vi "Process.vi"(8 "error in":errorcluster, 11 "Example Instrument UI":refnum<class "Instrument.PPMS2 UI.lvclass">) -> (0 "error out":errorcluster, 3 "Example Instrument UI out":refnum<class "Instrument.PPMS2 UI.lvclass">)   [LabVIEW 2016, in "Instrument.PPMS2 UI.lvclass"]
doc: "---------------------------------------------------------------\nJKI State Machine Objects™\nhttp://jki.net/state-machine-objects/\nCopyright (C) 2005-2015, JKI <info@jki.net>\nALL RIGHTS RESERVEDJKI State Machine Objects (SMO) 1.0.0.5\nJKI - JKI\nCopyright (c) 2016, JKI"
uses:
  Instrument.PPMS2 UI.lvclass
  C:/Program Files (x86)/National Instruments/LabVIEW 2016/vi.lib/JKI/JKI SMO/SMO/SMO.lvclass
  C:/Program Files (x86)/National Instruments/LabVIEW 2016/vi.lib/JKI/JKI SMO/SMO.UI/SMO.UI.lvclass
  instrument.PPMS2/Typedefs/Magnet Status--PPMS2--ring.ctl
  instrument.PPMS2/Typedefs/Temperature Status--PPMS2--ring.ctl
  <vilib>/JKI/JKI SMO/SMO/Typedefs/Parent Call--Enum.ctl
  instrument.PPMS2/instrument.PPMS2.lvclass
  C:/Program Files (x86)/National Instruments/LabVIEW 2016/user.lib/LevyLab/Levylab Instruments/SMOs/Instrument/Instrument.lvclass
  Instrument.PPMS2 UI.lvclass/Instrument.PPMS2 UI.ctl
  instrument.PPMS2/Typedefs/getAll--PPMS2--cluster.ctl
  <vilib>/JKI/JKI SMO/SMO.UI/SMO.UI.lvclass
  <vilib>/JKI/JKI SMO/SMO/SMO.lvclass
  <userlib>/LevyLab/Levylab Instruments/SMOs/Instrument/Instrument.lvclass
panel:
  in  "Angle":bool
  in  "Field":bool
  in  "Temperature":bool
  in  "Target Angle (°)":dbl=-0.00643419474363327 format="%_3g"
  in  "Target Field (Oe)":dbl=-0.00643419474363327 format="%_3g"
  in  "Target Temperature (K)":dbl=305.0156 format="%#_5g"
  out "PPMS 2 Temperature Status":T1 items=["TemperatureUnknown"=0, "Stable"=1, "Tracking"=2, "Near"=5, "Chasing"=6, "Filling"=7, "Standby"=10, "Disabled"=13, "ImpedanceNotFunction"=14, "TempFailure"=15]
  out "PPMS 2 Magnet Status":T2=1 items=["MagnetUnknown"=0, "StablePersistent"=1, "WarmingSwitch"=2, "CoolingSwitch"=3, "StableDriven"=4, "Iterating"=5, "Charging"=6, "Discharging"=7, "CurrentError"=8, "MagnetFailure"=15]
  out "Helium Level (%)":dbl=86.7
  out "Position (°)":dbl=90.002
  out "Field (Oe)":dbl=-0.00643419474363327 format="%_3g"
  out "Temperature(K)":dbl=305.0156 format="%#_5g"
  in  "update time (ms)":u32=200
  in  "STOP":bool
  # "PPMS 2 Monitor"
  # "SMO UI Template"
  # "For instructions on how to use the JKI State Machine Objects, examples and video tutorials, visit:\nhttp://jki.net/state-machine-objects/\n\nJKI State Machine Objects™\nhttp://jki.net/state-machine-objects/\nCopyright (C) 2005-2015, JKI <info@jki.net>\nALL RIGHTS RESERVED"
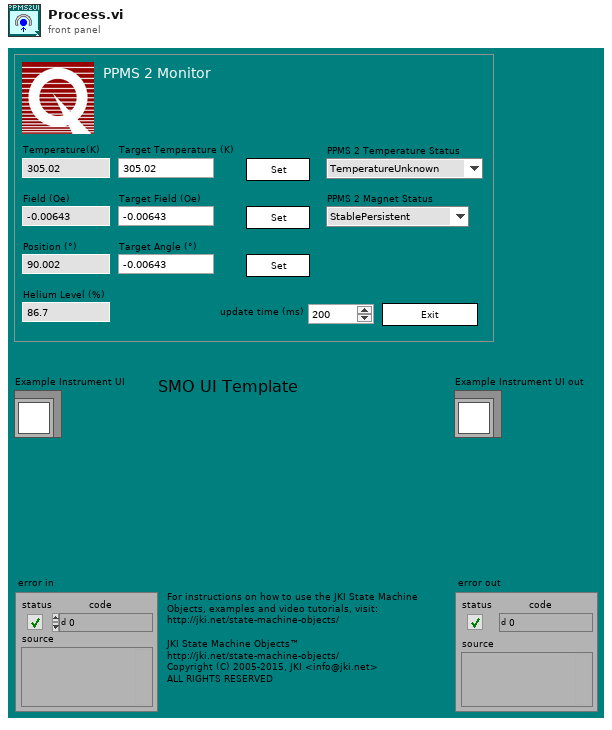
[diagram p1: front panel]
types:
  T1 = typedef "instrument.PPMS2.lvclass/Temperature Status--PPMS2--ring.ctl" = i32
  T2 = typedef "instrument.PPMS2.lvclass/Magnet Status--PPMS2--ring.ctl" = i32
  T3 = typedef "SMO.lvclass/Parent Call--Enum.ctl" = enum16{"Allows parent to run", "Does not request parent to run"}
  T4 = enum32{"invalid app kind", "Development System", "Run Time System", "Student Edition", "Embedded LabVIEW", "Evaluation", "Custom"}
  T5 = enum32{"Invalid", "Standard", "Closed", "Hidden", "Minimized", "Maximized"}
  T6 = typedef "instrument.PPMS2.lvclass/getAll--PPMS2--cluster.ctl" = cluster{"PPMS 2 Helium Level":dbl, "PPMS 2 Temperature":dbl, "PPMS 2 Temperature Status":T1, "PPMS 2 Magnetic Field":dbl, "PPMS 2 Magnet Status":T2, "PPMS 2 Position":dbl}
  T7 = cluster{"Core":cluster{"Current VI Reference":refnum<vi>, "Close Panel on Exit?":bool, "error":errorcluster}, "Self Reference":refnum<class "Instrument.PPMS2 UI.lvclass">, "instrument.PPMS2":refnum<class "instrument.PPMS2.lvclass">, "Data Send":variant, "Data Receive":variant}
  T8 = cluster{"Current VI Reference":refnum<vi>, "Close Panel on Exit?":bool, "error":errorcluster}
  T9 = typedef "SMO.lvclass/Protected Events.ctl" = cluster{"StopProcesses":refnum<user-event>, "AbortProcesses":refnum<user-event>, "Config Changed":refnum<user-event>, "Dependency":refnum<user-event>}
  T10 = typedef "Instrument.lvclass/PublicEvents--Cluster.ctl" = cluster{"MessageFromProcess":refnum<user-event>}
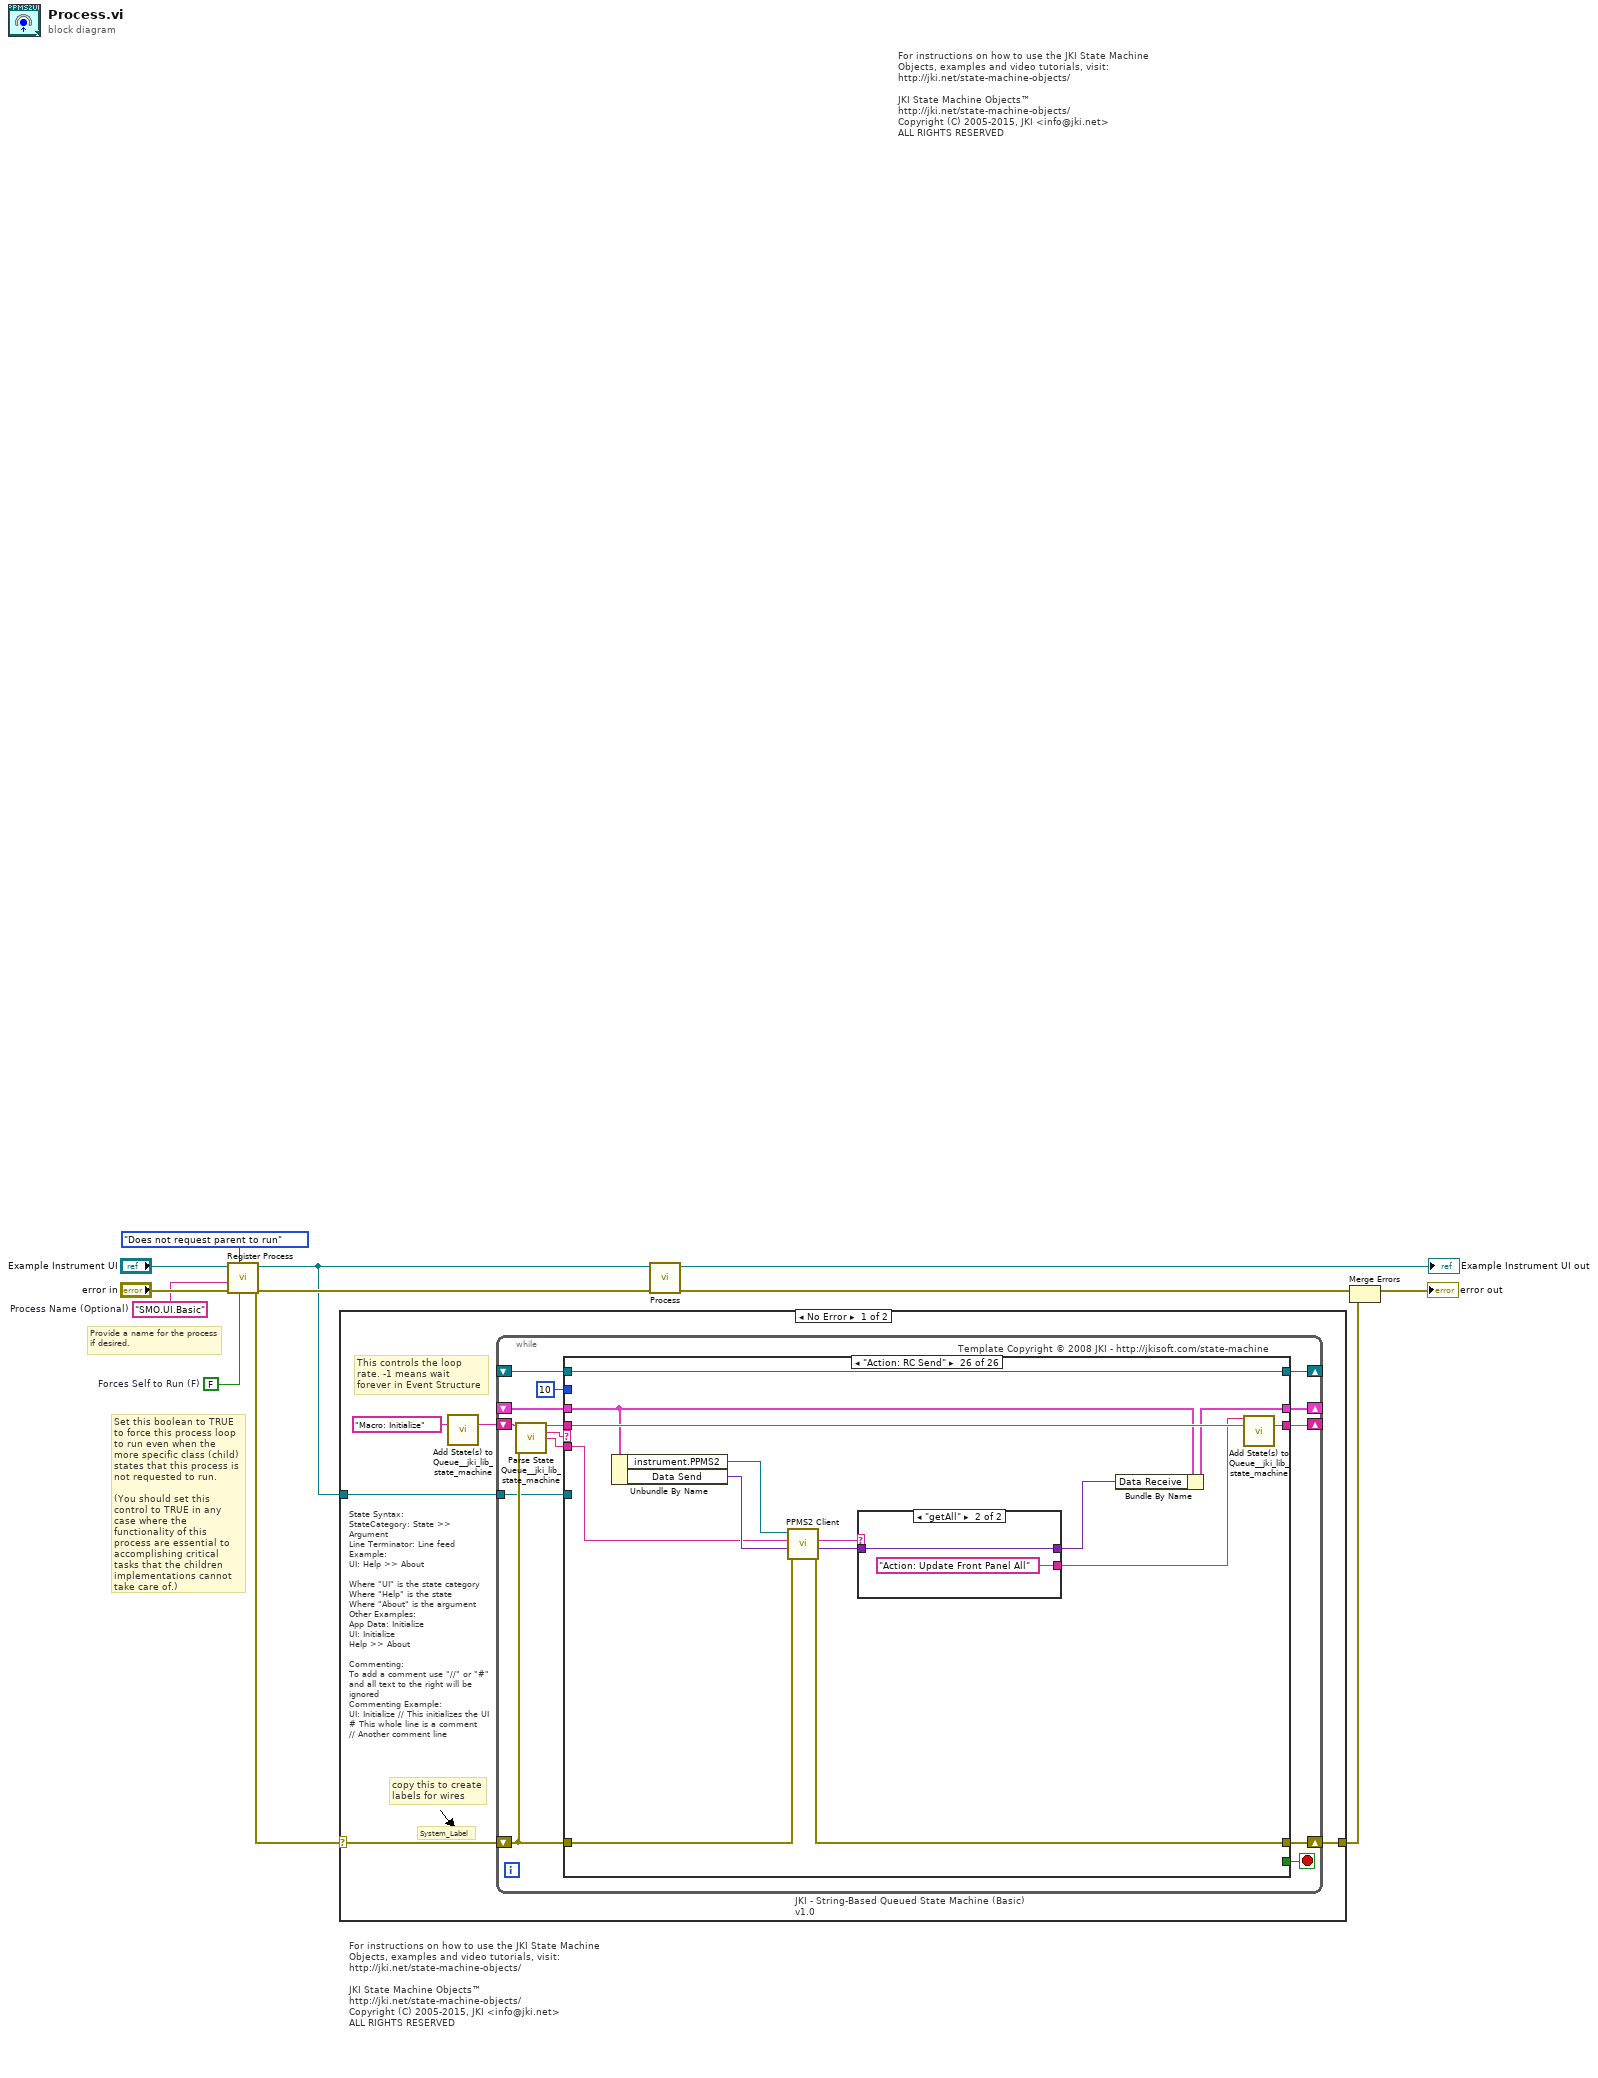
[diagram p0: block diagram]
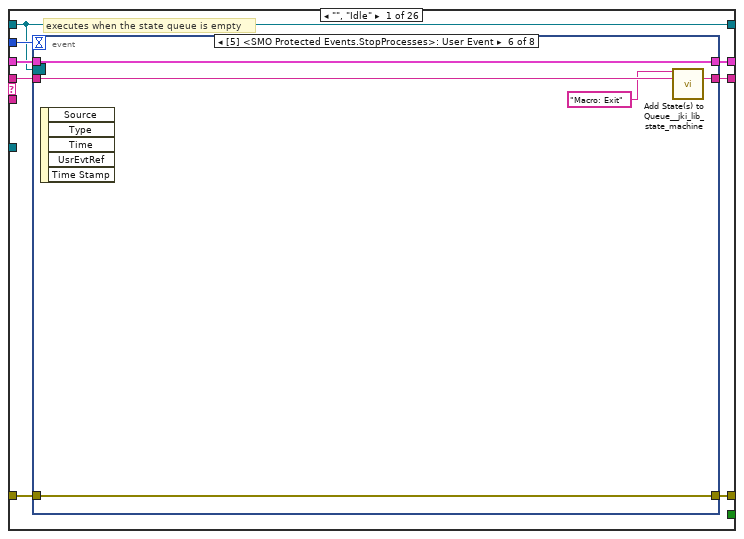
[diagram p2: hidden frame]
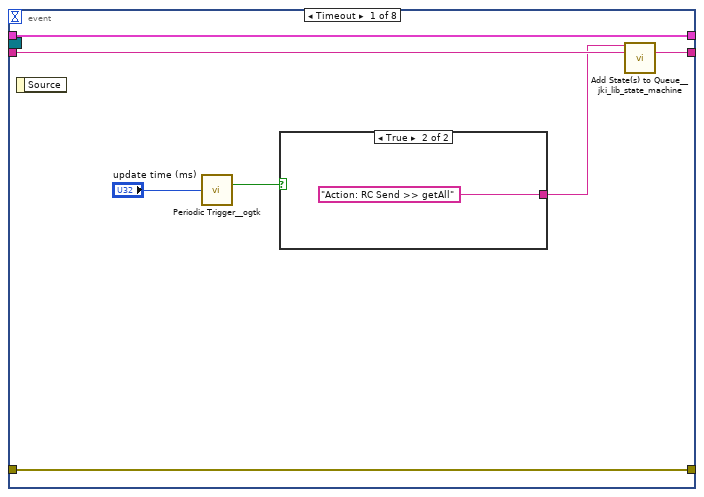
[diagram p3: hidden frame]
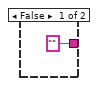
[diagram p4: hidden frame]
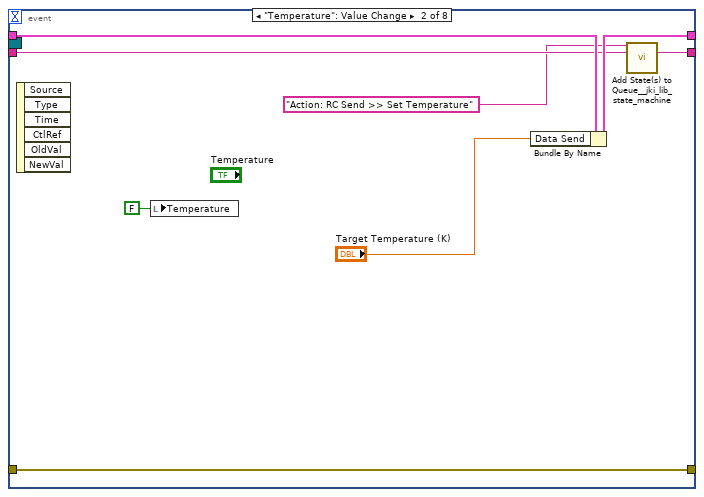
[diagram p5: hidden frame]
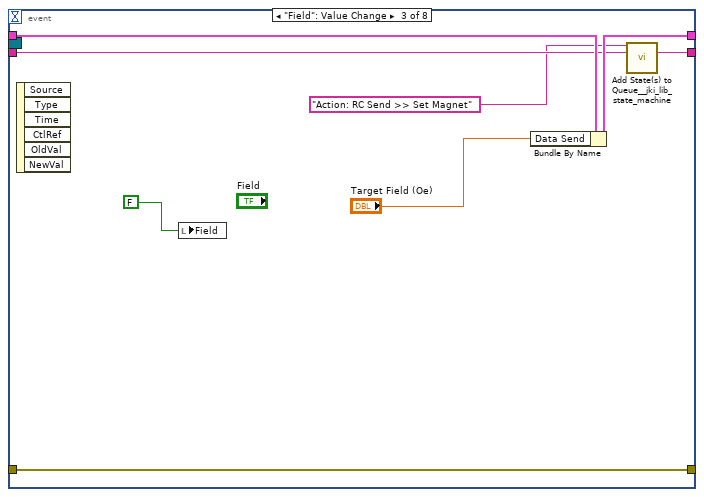
[diagram p6: hidden frame]
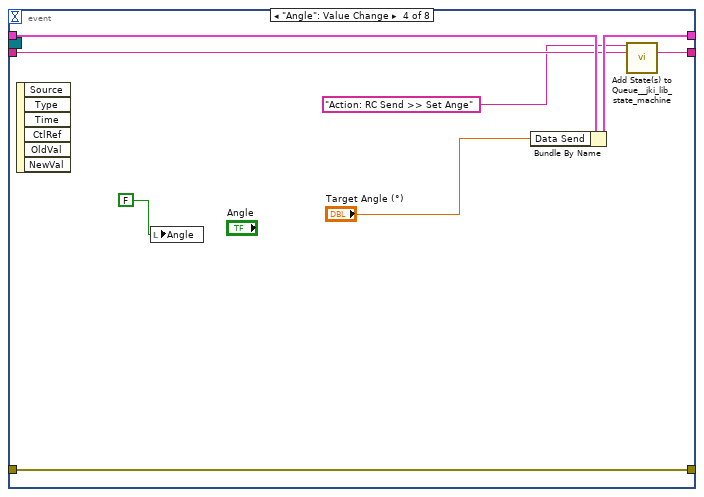
[diagram p7: hidden frame]
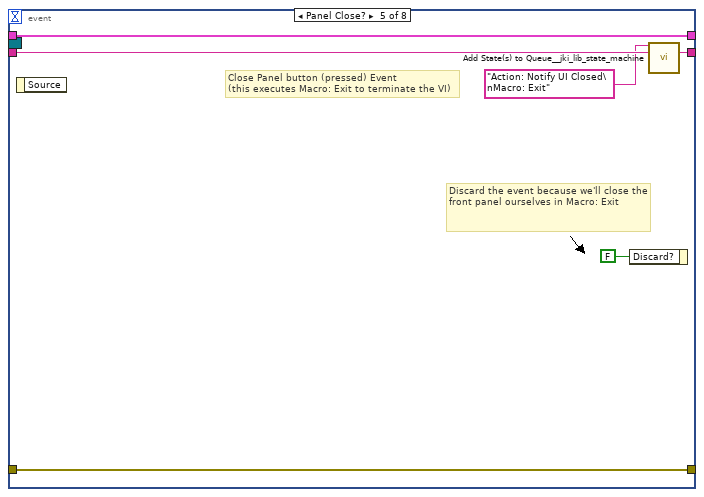
[diagram p8: hidden frame]
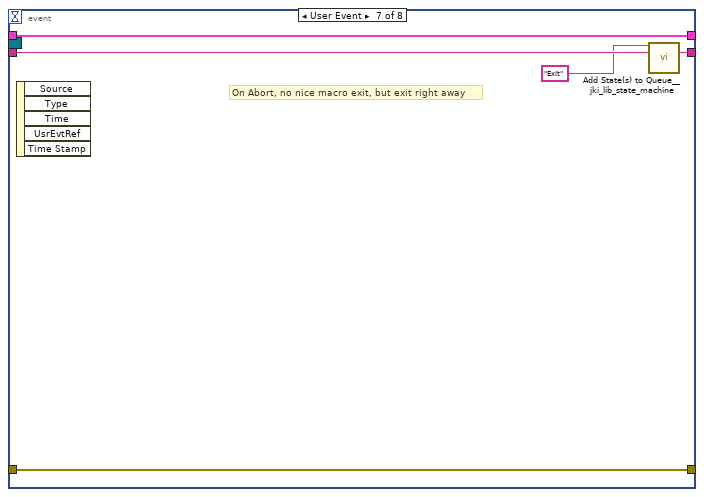
[diagram p9: hidden frame]
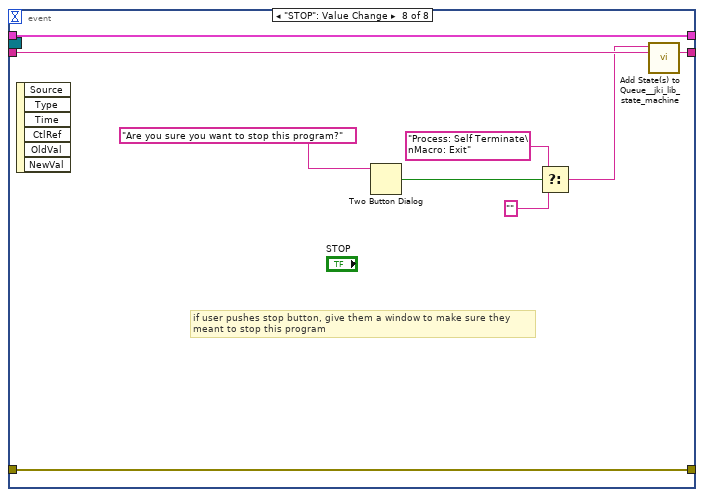
[diagram p10: hidden frame]
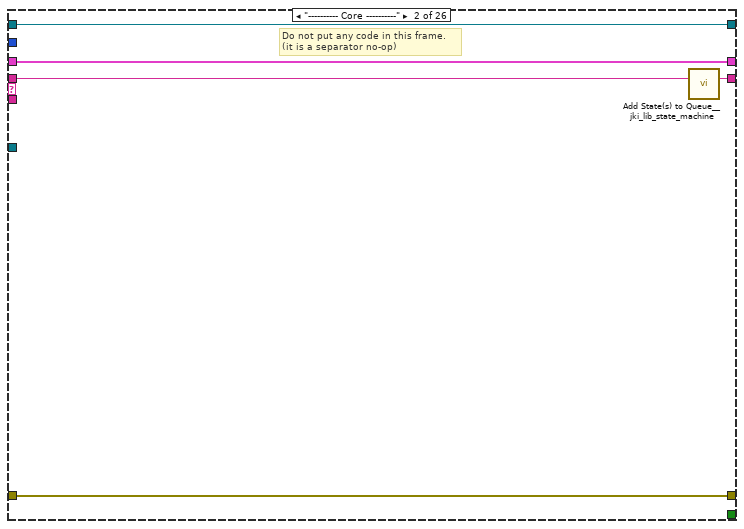
[diagram p11: hidden frame]
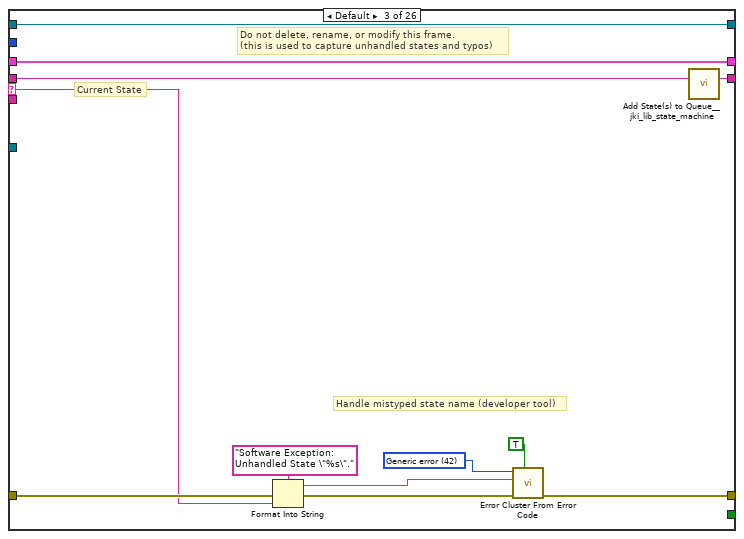
[diagram p12: hidden frame]
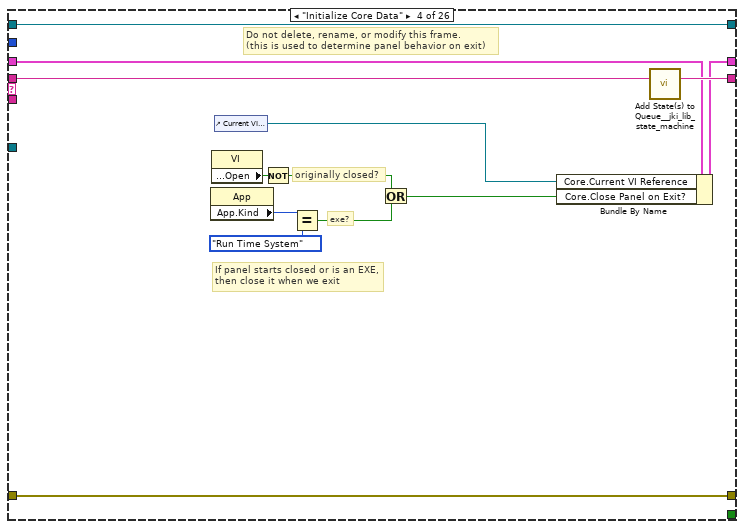
[diagram p13: hidden frame]
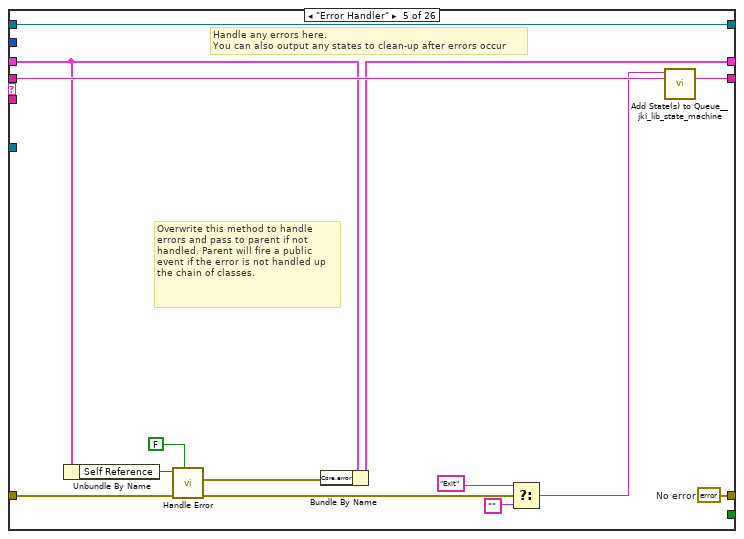
[diagram p14: hidden frame]
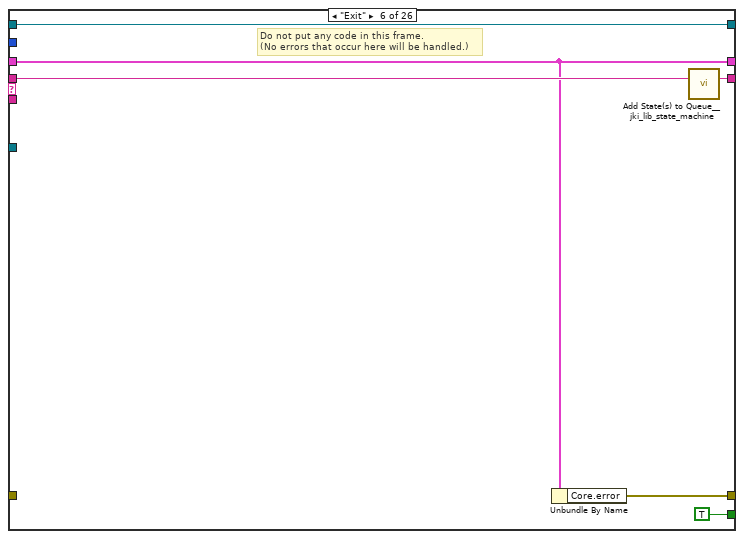
[diagram p15: hidden frame]
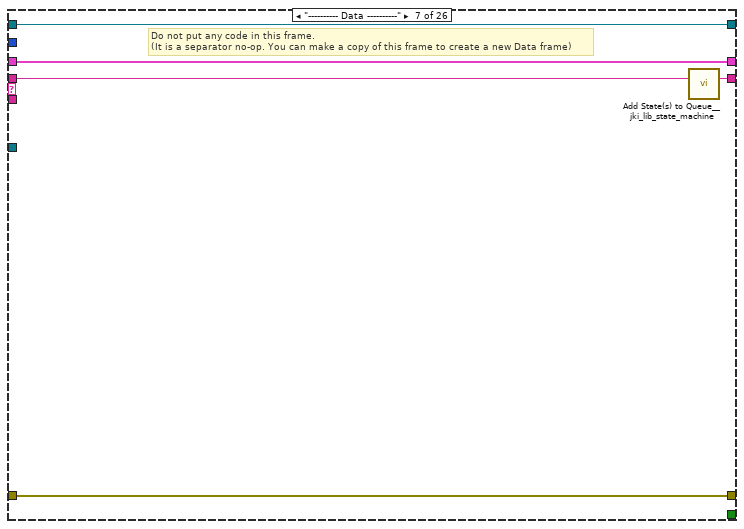
[diagram p16: hidden frame]
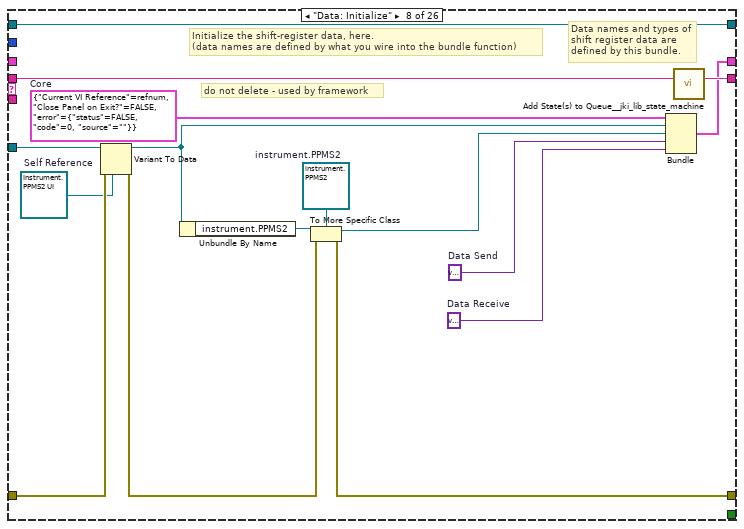
[diagram p17: hidden frame]
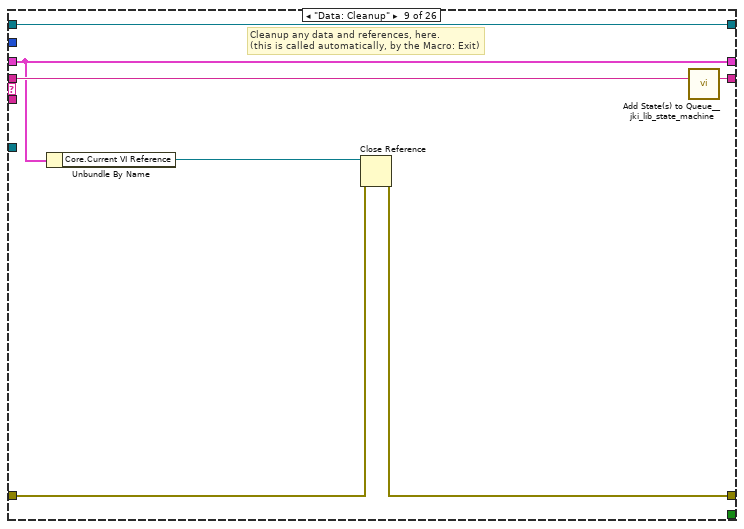
[diagram p18: hidden frame]
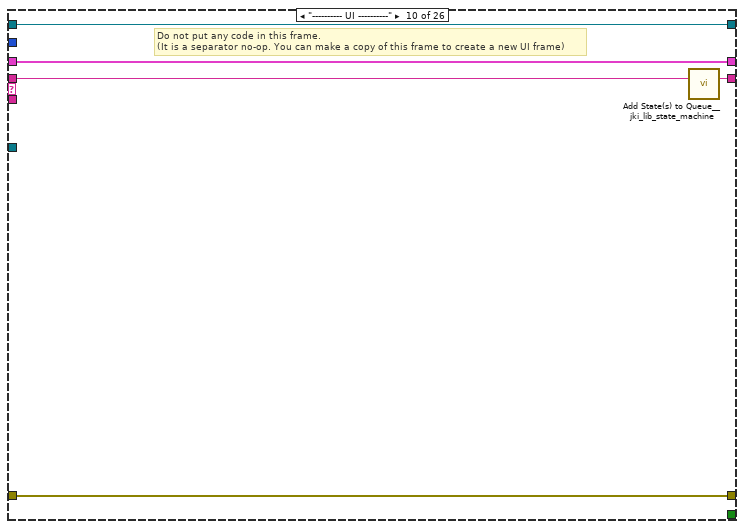
[diagram p19: hidden frame]
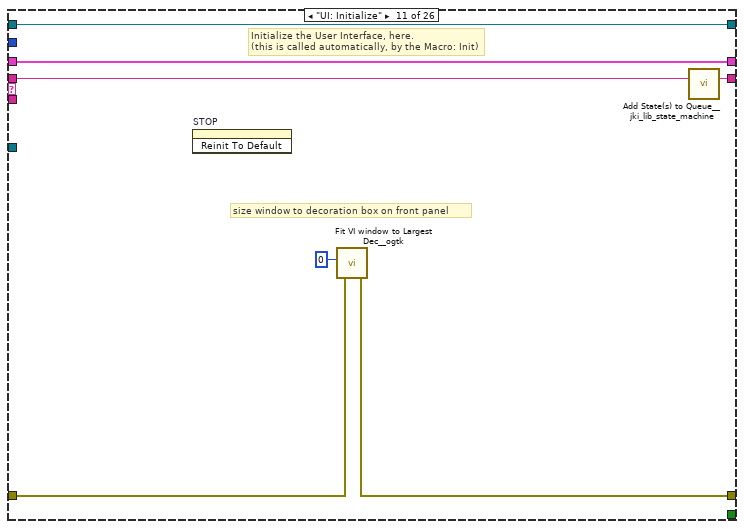
[diagram p20: hidden frame]
diagram:
  w2 = FALSE  # Forces Self to Run (F)
  w1 = "SMO.UI.Basic"  # Process Name (Optional)
  # "For instructions on how to use the JKI State Machine Objects, examples and video tutorials, visit:\nhttp://jki.net/state-machine-objects/\n\nJKI State Machine Objects™\nhttp://jki.net/state-machine-objects/\nCopyright (C) 2005-2015, JKI <info@jki.net>\nALL RIGHTS RESERVED"
  # "Provide a name for the process\nif desired."
  # "Set this boolean to TRUE to force this process loop to run even when the more specific class (child) states that this process is not requested to run.\n\n(You should set this control to TRUE in any case where the functionality of this process are essential to accomplishing critical tasks that the children implementations cannot take care of.)"
  # "For instructions on how to use the JKI State Machine Objects, examples and video tutorials, visit:\nhttp://jki.net/state-machine-objects/\n\nJKI State Machine Objects™\nhttp://jki.net/state-machine-objects/\nCopyright (C) 2005-2015, JKI <info@jki.net>\nALL RIGHTS RESERVED"
  n1 = call <vilib>:"Register Process.vi"("Forces Self to Run (F)"=w2, "Parent Call"=Parent_Call--Enum."Does not request parent to run", "error in (no error)"="error in", "Process Name (optional)"=w1, "SMO"="Example Instrument UI") -> ("error out"=w8:errorcluster, "SMO out"=w7:refnum<class "Instrument.PPMS2 UI.lvclass">)  [unwired: 5 in]
  n2 = case shown="No Error" w8 {
    selector: w8 -> [w13 w359]
    tunnel: w7 -> [w14 _]
    tunnel: [w12 w359] -> w4
    frame No Error {
      # "State Syntax:\nStateCategory: State >> Argument\nLine Terminator: Line feed\nExample:\nUI: Help >> About\n\nWhere \"UI\" is the state category\nWhere \"Help\" is the state\nWhere \"About\" is the argument\nOther Examples:\nApp Data: Initialize\nUI: Initialize\nHelp >> About\n\nCommenting:\nTo add a comment use \"//\" or \"#\" and all text to the right will be ignored\nCommenting Example:\nUI: Initialize // This initializes the UI\n# This whole line is a comment\n// Another comment line"
      # "copy this to create labels for wires"
      # "This controls the loop rate. -1 means wait forever in Event Structure"
      # "System_Label"
      n3 = call <vilib>:"Add State(s) to Queue__jki_lib_state_machine.vi"("State(s) in (\"\")"="Macro: Initialize") -> ("States Out"=w16:string)  [unwired: 14 in]
      n4 = while "JKI - String-Based Queued State Machine (Basic) v1.0" {
        shift-right: [w23] -> _
        shift-left: _ -> [w22]
        shift-right: [w26] -> w12
        shift-left: w13 -> [w20]
        shift-right: [w25] -> _
        shift-left: w16 -> [w27]
        tunnel: w14 -> [w19]
        shift-right: [w18] -> _
        shift-left: _ -> [w17]
        stop <- w24 stop-if-true
        # "Template Copyright © 2008 JKI - http://jkisoft.com/state-machine"
        n5 = call <vilib>:"Parse State Queue__jki_lib_state_machine.vi"("State Queue"=w27, "Error In (no error)"=w20) -> ("Remaining States"=w29:string, "Current State"=w30:string, "Arguments"=w28:string)  [unwired: 11 in]
        n6 = case shown="\"Action: RC Send\"" w30 {
          selector: w30 -> [_ _ w103 _ _ _ _ _ _ _ _ _ _ _ _ _ _ _ _ _ _ _ _ _ _ _]
          tunnel: w29 -> [w38 w101 w107 w126 w140 w146 w151 w167 w174 w179 w186 w193 w209 w241 w250 w264 w269 w280 w287 w292 w305 w311 w318 w325 w340 w354]
          tunnel: w28 -> [_ _ _ _ _ _ _ _ _ _ _ w187 w203 _ _ _ _ _ _ _ _ _ _ _ _ w346]
          tunnel: w22 -> [w36 w98 w105 w117 w128 w142 w148 _ w170 w176 w184 w191 w205 w238 w246 w255 w266 w277 w282 w289 w303 w309 w314 w321 w337 w351]
          tunnel: [w35 w99 w109 w123 w133 w141 w149 w153 w171 w177 w181 w188 w206 w239 w248 w262 w267 w271 w283 w290 w298 w306 w315 w319 w335 w344] -> w26
          tunnel: w20 -> [w34 w99 w108 w123 w129 _ w149 w164 w168 w177 w182 w189 w207 w239 w248 w262 w267 w272 w284 w290 w300 w307 w315 w320 w336 w345]
          tunnel: [w37 w100 w106 w125 w139 w145 w150 w166 w173 w178 w185 w192 w208 w240 w249 w263 w268 w279 w286 w291 w304 w310 w317 w324 w339 w353] -> w25
          tunnel: [_ _ _ _ _ TRUE _ _ _ _ _ _ _ _ _ _ _ _ _ _ _ _ _ _ _ _] -> w24
          tunnel: [w33 w98 w105 w124 w131 w142 w148 w165 w170 w176 w184 w191 w205 w238 w246 w255 w266 w277 w282 w289 w303 w309 w313 w321 w337 w350] -> w23
          tunnel: 10 ("Timeout") -> [w32 _ _ _ _ _ _ _ _ _ _ _ _ _ _ _ _ _ _ _ _ _ _ _ _ _]
          tunnel: w19 -> [_ _ _ _ _ _ _ w162 _ _ _ _ _ _ _ _ _ _ _ _ _ _ _ _ _ _]
          tunnel: [w31 w97 w102 w114 w138 w143 w147 w161 w169 w175 w183 w190 w202 w237 w247 w256 w265 w278 w285 w288 w302 w308 w316 w323 w338 w352] -> w18
          tunnel: w17 -> [w31 w97 w102 w114 w138 w143 w147 w161 w169 w175 w183 w190 w202 w237 w247 w256 w265 w278 w285 w288 _ w308 w316 w323 w338 w352]
          frame "", "Idle" {
            # "executes when the state queue is empty"
            n7 = event shown="[5] <SMO Protected Events.StopProcesses>: User Event" {
              selector: w31 -> [_ _ _ _ _ _ _ _]
              dyn-events: _ -> [_ _ _ _ _ _ _ _]
              timeout: w32 -> [_ _ _ _ _ _ _ _]
              tunnel: w38 -> [w45 w51 w59 w67 w77 w82 w87 w96]
              tunnel: [w44 w54 w62 w70 w76 w81 w86 w95] -> w37
              tunnel: w36 -> [w42 w53 w61 w69 w73 w79 w84 w93]
              tunnel: [w43 w55 w63 w71 w72 w80 w85 w94] -> w35
              tunnel: w34 -> [w43 w55 w63 w71 w72 w80 w85 w94]
              tunnel: [w42 w52 w60 w68 w73 w79 w84 w93] -> w33
              event Timeout {
                n8 = event-data() -> ()  [unwired: 1 in, 1 out]
                n9 = call <userlib>:"Periodic Trigger__ogtk.vi"("time (ms)"="update time (ms)") -> ("Triggered"=w41:bool)  [unwired: 12 in, 2 out]
                n10 = case shown="True" w41 {
                  tunnel: ["" "Action: RC Send >> getAll"] -> w39
                  frame False {
                  }
                  frame True {
                  }
                }
                n11 = call <vilib>:"Add State(s) to Queue__jki_lib_state_machine.vi"("State(s) in Front (\"\")"=w39, "State(s) in (\"\")"=w45) -> ("States Out"=w44:string)  [unwired: 13 in]
              }
              event "Temperature": Value Change {
                n12 = event-data() -> ()  [unwired: 1 in, 6 out]
                n13 = local write "Temperature"(FALSE ("Temperature")) -> ()
                n14 = Bundle By Name(cluster=w53, "Data Send"="Target Temperature (K)") -> (w52:T7)
                n15 = call <vilib>:"Add State(s) to Queue__jki_lib_state_machine.vi"("State(s) in Front (\"\")"="Action: RC Send >> Set Temperature" ("State(s) in Front (\"\")"), "State(s) in (\"\")"=w51) -> ("States Out"=w54:string)  [unwired: 13 in]
              }
              event "Field": Value Change {
                n16 = event-data() -> ()  [unwired: 1 in, 6 out]
                n17 = local write "Field"(FALSE ("Field")) -> ()
                n18 = Bundle By Name(cluster=w61, "Data Send"="Target Field (Oe)") -> (w60:T7)
                n19 = call <vilib>:"Add State(s) to Queue__jki_lib_state_machine.vi"("State(s) in Front (\"\")"="Action: RC Send >> Set Magnet" ("State(s) in Front (\"\")"), "State(s) in (\"\")"=w59) -> ("States Out"=w62:string)  [unwired: 13 in]
              }
              event "Angle": Value Change {
                n20 = event-data() -> ()  [unwired: 1 in, 6 out]
                n21 = local write "Angle"(FALSE ("Angle")) -> ()
                n22 = Bundle By Name(cluster=w69, "Data Send"="Target Angle (°)") -> (w68:T7)
                n23 = call <vilib>:"Add State(s) to Queue__jki_lib_state_machine.vi"("State(s) in Front (\"\")"="Action: RC Send >> Set Ange" ("State(s) in Front (\"\")"), "State(s) in (\"\")"=w67) -> ("States Out"=w70:string)  [unwired: 13 in]
              }
              event Panel Close? {
                # "Discard the event because we'll close the front panel ourselves in Macro: Exit"
                # "Close Panel button (pressed) Event\n(this executes Macro: Exit to terminate the VI)"
                n24 = event-data() -> ()  [unwired: 1 in, 1 out]
                n25 = event-data("Discard?"=FALSE) -> ()  [unwired: 1 in, 1 out]
                n26 = call <vilib>:"Add State(s) to Queue__jki_lib_state_machine.vi"("State(s) in Front (\"\")"="Action: Notify UI Closed\nMacro: Exit", "State(s) in (\"\")"=w77) -> ("States Out"=w76:string)  [unwired: 13 in]
              }
              event User Event {
                n27 = event-data() -> ()  [unwired: 1 in, 5 out]
                n28 = call <vilib>:"Add State(s) to Queue__jki_lib_state_machine.vi"("State(s) in Front (\"\")"="Macro: Exit", "State(s) in (\"\")"=w82) -> ("States Out"=w81:string)  [unwired: 13 in]
              }
              event User Event {
                # "On Abort, no nice macro exit, but exit right away"
                n29 = event-data() -> ()  [unwired: 1 in, 5 out]
                n30 = call <vilib>:"Add State(s) to Queue__jki_lib_state_machine.vi"("State(s) in Front (\"\")"="Exit", "State(s) in (\"\")"=w87) -> ("States Out"=w86:string)  [unwired: 13 in]
              }
              event "STOP": Value Change {
                # "if user pushes stop button, give them a window to make sure they\nmeant to stop this program"
                n31 = event-data() -> ()  [unwired: 1 in, 6 out]
                n32 = Two Button Dialog(message="Are you sure you want to stop this program?") -> (T button?=w92:bool)  [unwired: 2 in]
                n33 = Select(t="Process: Self Terminate\nMacro: Exit", s=w92, f="") -> (s? t:f=w88:string)
                n34 = call <vilib>:"Add State(s) to Queue__jki_lib_state_machine.vi"("State(s) in Front (\"\")"=w88, "State(s) in (\"\")"=w96) -> ("States Out"=w95:string)  [unwired: 13 in]
              }
            }
          }
          frame "---------- Core ----------" {
            # "Do not put any code in this frame.\n(it is a separator no-op)"
            n35 = call <vilib>:"Add State(s) to Queue__jki_lib_state_machine.vi"("State(s) in (\"\")"=w101) -> ("States Out"=w100:string)  [unwired: 14 in]
          }
          frame Default {
            w112 = 42 items=["No error", "Argument error", "Memory is full", "Out of zone", "End of file", "File already open", "Generic file I/O error", "File not found", "File permission error", "Disk is full", "Duplicate path", "Too many files open", "System feature not enabled", "Resource file not found", "Cannot add resource", "Resource not found", "Image not found", "Image memory error", "Pen does not exist", "Config type invalid", "Config token not found", "Config parse error", "Config memory error", "Bad external code format", "Bad external code offset", "External code not present", "Null window", "Destroy window error", "Null menu", "Print aborted", "Bad print record", "Print driver error", "Windows error during printing", "Memory error during printing", "Print dialog error", "Generic print error", "Invalid device refnum", "Device not found", "Device parameter error", "Device unit error", "Cannot open device", "Device call aborted", "Generic error", "Cancelled by user", "Object ID too low", "Object ID too high", "Object not in heap", "Unknown heap", "Unknown object (invalid DefProc)", "Unknown object (DefProc not in table)", "Message out of range", "Invalid (null) method", "Unknown message", "Manager call not supported", "Bad address", "Network operation in progress", "Network operation timed out", "Connection is busy", "Network attribute not supported", "Network error", "Address in use", "System out of memory", "Connection aborted", "Connection refused", "Not connected", "Already connected", "Connection closed", "Initialization error (interapplication manager)", "Bad occurrence", "Wait on unbound occurrence handler", "Occurrence queue overflow", "Datalog type conflict", "Unused", "Unrecognized type (interapplication manager)", "Memory corrupt", "Failed to make temporary DLL", "Old CIN version", "Drag socket not found", "Failed to load drop-object", "Failed to register OLE object", "Failed to release OLE object", "Format specifier type mismatch", "Unknown format specifier", "Too few format specifiers", "Too many format specifiers", "Scan failed", "Newer CIN version", "Error converting to variant", "Runtime menu error", "Password tampered", "Variant attribute not found", "Incompatible variant data type", "Event data is not available", "Event Store is not present", "Occurrence is not found", "Event Queue is not created", "Event info is not available", "Refnum passed is NULL", "Error retrieving Class GUID", "Error retrieving CoClass GUID", "Error retrieving TypeLib GUID.", "Bad built application magic bytes.", "Specific driver is different from the specific driver associated with the Logical Name.", "There is no session opened to the class driver.", "Max Error", "MAX - Error with config objects", "MAX - Error loading configuration", "MAX - Group not supported"]
            # "Current State"
            # "Do not delete, rename, or modify this frame.\n(this is used to capture unhandled states and typos)"
            # "Handle mistyped state name (developer tool)"
            n36 = Format Into String(format string="Software Exception: Unhandled State \"%s\"." ("message"), error in=w108, w103) -> (resulting string=w111:string, error out=w110:errorcluster)  [unwired: 1 in]
            n37 = call <vilib>:"Error Cluster From Error Code.vi"("show call chain? (False)"=TRUE, "error in (no error)"=w110, "error message (\"\")"=w111, "error code (0)"=w112) -> ("error out"=w109:errorcluster)  [unwired: 5 in]
            n38 = call <vilib>:"Add State(s) to Queue__jki_lib_state_machine.vi"("State(s) in (\"\")"=w107) -> ("States Out"=w106:string)  [unwired: 14 in]
          }
          frame "Initialize Core Data" {
            # "Do not delete, rename, or modify this frame.\n(this is used to determine panel behavior on exit)"
            # "originally closed?"
            # "exe?"
            # "If panel starts closed or is an EXE, then close it when we exit"
            n39 = property class="App"() -> ("App.Kind"=w121:T4)  [unwired: 2 in, 2 out]
            n40 = property class="VI"() -> ("Front Panel.Open"=w122:bool)  [unwired: 2 in, 2 out]
            n41 = control-ref of="Current VI Reference"() -> (w115:refnum<vi>)
            n42 = Not(x=w122) -> (.not. x?=w119:bool)
            n43 = Equal?(x=w121, y=T4."Run Time System" ("Application:Kind")) -> (x = y?=w118:bool)
            n44 = Or(x=w119, y=w118) -> (x .or. y?=w116:bool)
            n45 = Bundle By Name(cluster=w117, "Core.Current VI Reference"=w115, "Core.Close Panel on Exit?"=w116) -> (w124:T7)
            n46 = call <vilib>:"Add State(s) to Queue__jki_lib_state_machine.vi"("State(s) in (\"\")"=w126) -> ("States Out"=w125:string)  [unwired: 14 in]
          }
          frame "Error Handler" {
            w133 = errorcluster {"status"=FALSE, "code"=0, "source"=""}  # No error
            # "Overwrite this method to handle errors and pass to parent if not handled. Parent will fire a public event if the error is not handled up the chain of classes."
            # "Handle any errors here.\nYou can also output any states to clean-up after errors occur"
            n47 = Unbundle By Name(w128) -> ("Self Reference"=w137:refnum<class "Instrument.PPMS2 UI.lvclass">)
            n48 = call-dynamic "Handle Error.vi"("Stop on Unhandled Error (T)"=FALSE, "error in"=w129, "SMO"=w137) -> ("handling error"=w127:errorcluster, "Unhandled error"=w132:errorcluster)  [unwired: 6 in, 1 out]
            n49 = Bundle By Name(cluster=w128, "Core.error"=w132) -> (w131:T7)
            n50 = Select(t="Exit", s=w127, f="") -> (s? t:f=w134:string)
            n51 = call <vilib>:"Add State(s) to Queue__jki_lib_state_machine.vi"("State(s) in Front (\"\")"=w134, "State(s) in (\"\")"=w140) -> ("States Out"=w139:string)  [unwired: 13 in]
          }
          frame "Exit" {
            # "Do not put any code in this frame.\n(No errors that occur here will be handled.)"
            n52 = Unbundle By Name(w142) -> ("Core.error"=w141:errorcluster)
            n53 = call <vilib>:"Add State(s) to Queue__jki_lib_state_machine.vi"("State(s) in (\"\")"=w146) -> ("States Out"=w145:string)  [unwired: 14 in]
          }
          frame "---------- Data ----------" {
            # "Do not put any code in this frame.\n(It is a separator no-op. You can make a copy of this frame to create a new Data frame)"
            n54 = call <vilib>:"Add State(s) to Queue__jki_lib_state_machine.vi"("State(s) in (\"\")"=w151) -> ("States Out"=w150:string)  [unwired: 14 in]
          }
          frame "Data: Initialize" {
            w152 = variant  # Data Receive
            w157 = refnum<class "instrument.PPMS2.lvclass"> refnum  # instrument.PPMS2
            w158 = variant  # Data Send
            w160 = T8 {"Current VI Reference"=refnum, "Close Panel on Exit?"=FALSE, "error"={"status"=FALSE, "code"=0, "source"=""}}  # Core
            w163 = refnum<class "Instrument.PPMS2 UI.lvclass"> refnum  # Self Reference
            # "do not delete - used by framework"
            # "Data names and types of shift register data are defined by this bundle."
            # "Initialize the shift-register data, here.\n(data names are defined by what you wire into the bundle function)"
            n55 = Variant To Data(error in=w164, type=w163, Variant=w162) -> (data=w159:refnum<class "Instrument.PPMS2 UI.lvclass">, error out=w154:errorcluster)
            n56 = Unbundle By Name(w159) -> ("instrument.PPMS2"=w156:refnum<class "instrument.PPMS2.lvclass">)
            n57 = To More Specific Class(target class=w157, reference=w156, error in=w154) -> (specific class reference=w155:refnum<class "instrument.PPMS2.lvclass">, error out=w153:errorcluster)
            n58 = Bundle("Core"=w160, "Self Reference"=w159, "instrument.PPMS2"=w155, "Data Send"=w158, "Data Receive"=w152) -> (w165:T7)  [unwired: 1 in]
            n59 = call <vilib>:"Add State(s) to Queue__jki_lib_state_machine.vi"("State(s) in (\"\")"=w167) -> ("States Out"=w166:string)  [unwired: 14 in]
          }
          frame "Data: Cleanup" {
            # "Cleanup any data and references, here.\n(this is called automatically, by the Macro: Exit)"
            n60 = Unbundle By Name(w170) -> ("Core.Current VI Reference"=w172:refnum<vi>)
            n61 = Close Reference(reference=w172, error in (no error)=w168) -> (error out=w171:errorcluster)
            n62 = call <vilib>:"Add State(s) to Queue__jki_lib_state_machine.vi"("State(s) in (\"\")"=w174) -> ("States Out"=w173:string)  [unwired: 14 in]
          }
          frame "---------- UI ----------" {
            # "Do not put any code in this frame.\n(It is a separator no-op. You can make a copy of this frame to create a new UI frame)"
            n63 = call <vilib>:"Add State(s) to Queue__jki_lib_state_machine.vi"("State(s) in (\"\")"=w179) -> ("States Out"=w178:string)  [unwired: 14 in]
          }
          frame "UI: Initialize" {
            # "size window to decoration box on front panel"
            # "Initialize the User Interface, here.\n(this is called automatically, by the Macro: Init)"
            n64 = invoke on="STOP" class="Bool (strict)" method="Reinit To Default"() -> ()  [unwired: 3 in, 3 out]
            n65 = call <userlib>:"Fit VI window to Largest Dec__ogtk.vi"("error in (no error)"=w182, "border spacing (2 px)"=0) -> ("error out"=w181:errorcluster)  [unwired: 4 in, 1 out]
            n66 = call <vilib>:"Add State(s) to Queue__jki_lib_state_machine.vi"("State(s) in (\"\")"=w186) -> ("States Out"=w185:string)  [unwired: 14 in]
          }
          frame "UI: Cursor Set" {
            # "Argument"
            # "Initialize the User Interface, here.\n(this is called automatically, by the Macro: Init)"
            n67 = disable-structure shown="Default" {
              disable-tunnel: w189 -> [w194 w197]
              disable-tunnel: [w194 w196] -> w188
              disable-tunnel: w187 -> [_ w195]
              frame condition #0 {
              }
              frame condition #1 (active) {
                n68 = case shown="\"Busy\"" w195 {
                  tunnel: w197 -> [w199 w201]
                  tunnel: [w198 w200] -> w196
                  frame "Idle", Default {
                    n69 = call <vilib>:"Unset Busy.vi"("error in (no error)"=w199) -> ("error out"=w198:errorcluster)  [unwired: 10 in]
                  }
                  frame "Busy" {
                    n70 = call <vilib>:"Set Busy.vi"("error in (no error)"=w201) -> ("error out"=w200:errorcluster)  [unwired: 9 in, 1 out]
                  }
                }
              }
            }
            n71 = call <vilib>:"Add State(s) to Queue__jki_lib_state_machine.vi"("State(s) in (\"\")"=w193) -> ("States Out"=w192:string)  [unwired: 14 in]
          }
          frame "UI: Front Panel State" {
            # "Argument"
            # "Set Front Panel Open or Closed\n(Usage: \"UI: Front Panel State >> Open|Close\")"
            n72 = Unbundle By Name(w205) -> ("Core.Current VI Reference"=w204:refnum<vi>)
            n73 = disable-structure shown="Default" {
              disable-tunnel: w207 -> [w213 w236]
              disable-tunnel: [w212 w236] -> w206
              disable-tunnel: w204 -> [w211 _]
              disable-tunnel: w203 -> [w210 _]
              frame condition #0 (active) {
                n74 = case shown="\"Close\"" w210 {
                  tunnel: w213 -> [w217 w230]
                  tunnel: [w219 w231] -> w212
                  tunnel: w211 -> [w218 w228]
                  frame "Open", Default {
                    n75 = property class="VI"(reference=w218, error in=w217) -> (reference out=w215:refnum<vi>, error out=w216:errorcluster, "FP.State"=w214:T5)
                    n76 = case shown="\"Closed\"" w214 {
                      tunnel: [w222 w225] -> w219
                      tunnel: w216 -> [w221 w225]
                      tunnel: w215 -> [w220 _]
                      frame "Closed" {
                        n77 = invoke class="VI" method="FP.Open"(reference=w220, error in=w221, "Activate"=TRUE, "State"=T5."Standard") -> (error out=w222:errorcluster)  [unwired: 1 in, 4 out]
                      }
                      frame Default {
                      }
                    }
                  }
                  frame "Close" {
                    n78 = property class="VI"(reference=w228, error in=w230) -> (reference out=w227:refnum<vi>, error out=w229:errorcluster, "FP.State"=w226:T5)
                    n79 = case shown="Default" w226 {
                      tunnel: [w232 w235] -> w231
                      tunnel: w229 -> [w232 w234]
                      tunnel: w227 -> [_ w233]
                      frame "Invalid", "Closed" {
                      }
                      frame Default {
                        n80 = invoke class="VI" method="FP.Close"(reference=w233, error in=w234) -> (error out=w235:errorcluster)  [unwired: 1 in, 2 out]
                      }
                    }
                  }
                }
              }
              frame condition #1 {
              }
            }
            n81 = call <vilib>:"Add State(s) to Queue__jki_lib_state_machine.vi"("State(s) in (\"\")"=w209) -> ("States Out"=w208:string)  [unwired: 14 in]
          }
          frame "---------- Macro ----------" {
            # "Do not put any code in this frame.\n(It is a separator no-op. You can make a copy of this frame to create a new Macro frame)"
            n82 = call <vilib>:"Add State(s) to Queue__jki_lib_state_machine.vi"("State(s) in (\"\")"=w241) -> ("States Out"=w240:string)  [unwired: 14 in]
          }
          frame "Macro: Initialize" {
            # "Initialization Macro\n(This is called once, when the VI starts)"
            n83 = call <vilib>:"Add State(s) to Queue__jki_lib_state_machine.vi"("State(s) in Front (\"\")"="Data: Initialize\nInitialize Core Data\nEvents: Register", "State(s) in (\"\")"="Process: Sync", "State(s) at Back (\"\")"="UI: Initialize\nUI: Front Panel State >> Open") -> ("States Out"=w243:string)  [unwired: 12 in]
            n84 = call <vilib>:"Add State(s) to Queue__jki_lib_state_machine.vi"("State(s) in Front (\"\")"=w243, "State(s) in (\"\")"=w250) -> ("States Out"=w249:string)  [unwired: 13 in]
          }
          frame "Macro: Exit" {
            # "Exit Macro\n(This is called once, when the VI exits)"
            n85 = Unbundle By Name(w255) -> ("Core.Close Panel on Exit?"=w261:bool)
            n86 = Select(t="UI: Front Panel State >> Close", s=w261, f="") -> (s? t:f=w258:string)
            n87 = call <vilib>:"Add State(s) to Queue__jki_lib_state_machine.vi"("State(s) in Front (\"\")"="Data: Cleanup\nEvents: Unregister", "State(s) in (\"\")"="Process: Sync", "State(s) at Back (\"\")"="Exit") -> ("States Out"=w252:string)  [unwired: 12 in]
            n88 = call <vilib>:"Add State(s) to Queue__jki_lib_state_machine.vi"("State(s) in (\"\")"=w258, "State(s) at Back (\"\")"=w252) -> ("States Out"=w257:string)  [unwired: 13 in]
            n89 = call <vilib>:"Add State(s) to Queue__jki_lib_state_machine.vi"("State(s) in Front (\"\")"=w257, "State(s) in (\"\")"=w264) -> ("States Out"=w263:string)  [unwired: 13 in]
          }
          frame "---------- Process ----------" {
            # "Template Separator\n(You can make a copy of, or modify, this frame)"
            n90 = call <vilib>:"Add State(s) to Queue__jki_lib_state_machine.vi"("State(s) in (\"\")"=w269) -> ("States Out"=w268:string)  [unwired: 14 in]
          }
          frame "Process: Sync" {
            n91 = Unbundle By Name(w277) -> ("Self Reference"=w273:refnum<class "Instrument.PPMS2 UI.lvclass">)
            n92 = call <vilib>:"WaitOnProcessSync.vi"("error in (no error)"=w272, "SMO"=w273) -> ("error out"=w271:errorcluster, "Don't run?"=w276:bool)  [unwired: 7 in, 1 out]
            n93 = Select(t="Data: Cleanup\nEvents: Unregister\nExit", s=w276, f="") -> (s? t:f=w270:string)
            n94 = call <vilib>:"Add State(s) to Queue__jki_lib_state_machine.vi"("State(s) in Front (\"\")"=w270, "State(s) in (\"\")"=w280) -> ("States Out"=w279:string)  [unwired: 13 in]
          }
          frame "Process: Self Terminate" {
            n95 = Unbundle By Name(w282) -> ("Self Reference"=w281:refnum<class "Instrument.PPMS2 UI.lvclass">)
            n96 = call <vilib>:"SelfTerminate.vi"("error in (no error)"=w284, "SMO in"=w281) -> ("error out"=w283:errorcluster)  [unwired: 8 in, 1 out]
            n97 = call <vilib>:"Add State(s) to Queue__jki_lib_state_machine.vi"("State(s) in (\"\")"=w287) -> ("States Out"=w286:string)  [unwired: 14 in]
          }
          frame "---------- Events ----------" {
            # "Template Separator\n(You can make a copy of, or modify, this frame)"
            n98 = call <vilib>:"Add State(s) to Queue__jki_lib_state_machine.vi"("State(s) in (\"\")"=w292) -> ("States Out"=w291:string)  [unwired: 14 in]
          }
          frame "Events: Register" {
            # "Expand to add\nmore events"
            # "Base Class Protected Events"
            n99 = Unbundle By Name(w303) -> ("Self Reference"=w296:refnum<class "Instrument.PPMS2 UI.lvclass">, "instrument.PPMS2"=w295:refnum<class "instrument.PPMS2.lvclass">)
            n100 = call <vilib>:"GetProtectedEvents.vi"("SMO"=w296) -> ("error out"=w297:errorcluster, "SMO Protected Events"=w301:T9)  [unwired: 8 in, 1 out]
            n101 = call <userlib>:"Instrument.GetPublicEvents.vi"("Instrument"=w295) -> ("error out"=w293:errorcluster, "Instrument Public Events"=w294:T10)  [unwired: 8 in, 1 out]
            n102 = register-events(w301, w294) -> (reference out=w302:refnum<event-registration>, error out=w299:errorcluster)  [unwired: 2 in]
            n103 = Merge Errors(w293, w300, w299, w297) -> (w298:errorcluster)
            n104 = call <vilib>:"Add State(s) to Queue__jki_lib_state_machine.vi"("State(s) in (\"\")"=w305) -> ("States Out"=w304:string)  [unwired: 14 in]
          }
          frame "Events: Unregister" {
            n105 = Unregister For Events(event registration refnum=w308, error in=w307) -> (error out=w306:errorcluster)
            n106 = call <vilib>:"Add State(s) to Queue__jki_lib_state_machine.vi"("State(s) in (\"\")"=w311) -> ("States Out"=w310:string)  [unwired: 14 in]
          }
          frame "---------- Action ----------" {
            n107 = Unbundle By Name(w314) -> ("Self Reference"=w312:refnum<class "Instrument.PPMS2 UI.lvclass">)
            n108 = Bundle By Name(cluster=w314, "Self Reference"=w312) -> (w313:T7)
            n109 = call <vilib>:"Add State(s) to Queue__jki_lib_state_machine.vi"("State(s) in (\"\")"=w318) -> ("States Out"=w317:string)  [unwired: 14 in]
          }
          frame "Action: Notify UI Closed" {
            # "Notify that the UI has been closed"
            n110 = Unbundle By Name(w321) -> ("Self Reference"=w322:refnum<class "Instrument.PPMS2 UI.lvclass">)
            n111 = call <vilib>:"Hide.vi"("error in (no error)"=w320, "SMO.UI"=w322) -> ("error out"=w319:errorcluster)  [unwired: 8 in, 1 out]
            n112 = call <vilib>:"Add State(s) to Queue__jki_lib_state_machine.vi"("State(s) in (\"\")"=w325) -> ("States Out"=w324:string)  [unwired: 14 in]
          }
          frame "Action: Update Front Panel All" {
            n113 = Unbundle By Name(w337) -> ("Data Receive"=w334:variant)
            n114 = Variant To Data(error in=w336, type=T6 {"PPMS 2 Helium Level"=0.0, "PPMS 2 Temperature"=0.0, "PPMS 2 Temperature Status"=0, "PPMS 2 Magnetic Field"=0.0, "PPMS 2 Magnet Status"=1, "PPMS 2 Position"=0.0} ("getAll"), Variant=w334) -> (data=w332:T6, error out=w335:errorcluster)
            n115 = Unbundle By Name(w332) -> ("PPMS 2 Helium Level"=→"Helium Level (%)":dbl, "PPMS 2 Temperature"=→"Temperature(K)":dbl, "PPMS 2 Temperature Status"=→"PPMS 2 Temperature Status":T1, "PPMS 2 Magnetic Field"=→"Field (Oe)":dbl, "PPMS 2 Magnet Status"=→"PPMS 2 Magnet Status":T2, "PPMS 2 Position"=→"Position (°)":dbl)
            n116 = call <vilib>:"Add State(s) to Queue__jki_lib_state_machine.vi"("State(s) in (\"\")"=w340) -> ("States Out"=w339:string)  [unwired: 14 in]
          }
          frame "Action: RC Send" {
            n117 = Unbundle By Name(w351) -> ("instrument.PPMS2"=w341:refnum<class "instrument.PPMS2.lvclass">, "Data Send"=w347:variant)
            n118 = call "PPMS2 Client.vi"("error in (no error)"=w345, "Data"=w347, "Command"=w346, "instrument.PPMS2 in"=w341) -> ("error out"=w344:errorcluster, "Data out"=w343:variant, "Command out"=w342:string)  [unwired: 4 in, 1 out]
            n119 = case shown="\"getAll\"" w342 {
              tunnel: ["" "Action: Update Front Panel All"] -> w349
              tunnel: w343 -> [_ w357]
              tunnel: [variant ("Data") w357] -> w348
              frame Default {
              }
              frame "getAll" {
              }
            }
            n120 = Bundle By Name(cluster=w351, "Data Receive"=w348) -> (w350:T7)
            n121 = call <vilib>:"Add State(s) to Queue__jki_lib_state_machine.vi"("State(s) in Front (\"\")"=w349, "State(s) in (\"\")"=w354) -> ("States Out"=w353:string)  [unwired: 13 in]
          }
        }
      }
    }
    frame Error {
    }
  }
  n122 = call-parent "Process.vi"("error in (no error)"=w8, "SMO.UI"=w7) -> ("error out"=w5:errorcluster, "SMO.UI out"=→"Example Instrument UI out":refnum<class "Instrument.PPMS2 UI.lvclass">)  [unwired: 8 in]
  n123 = Merge Errors(w5, w4) -> (→"error out":errorcluster)
